vi "get_voltages.vi"(8 "error in (no error)":errorcluster, 11 "TrajectoryAK101022Resonance in":refnum<class "TrajectoryAK101022Resonance.lvclass">) -> (0 "error out":errorcluster, 1 "Vz min(V)":dbl, 2 "Vz max(V)":dbl, 3 "TrajectoryAK101022Resonance out":refnum<class "TrajectoryAK101022Resonance.lvclass">, 4 "Vy max(V)":dbl, 6 "Vy min(V)":dbl)   [LabVIEW 2010, in "TrajectoryAK101022Resonance.lvclass"]
uses:
  TrajectoryAK101022Resonance.lvclass
  TrajectoryAK101022Resonance.lvclass/TrajectoryAK101022Resonance.ctl
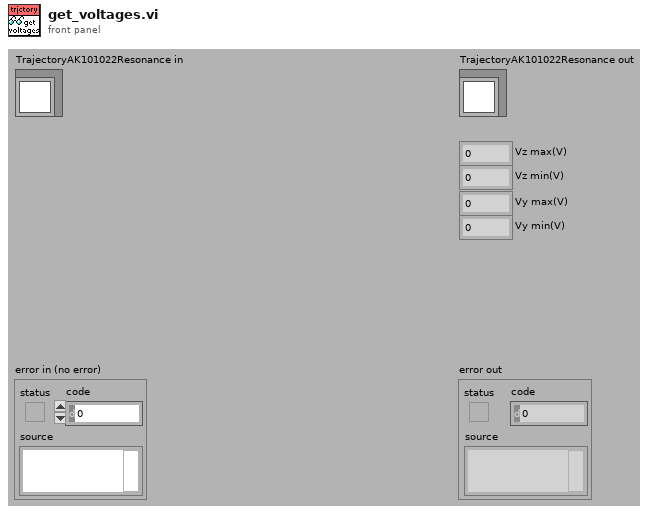
[diagram p1: front panel]
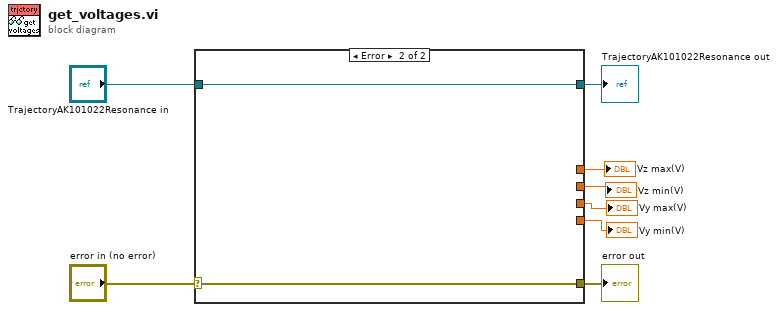
[diagram p0: block diagram]
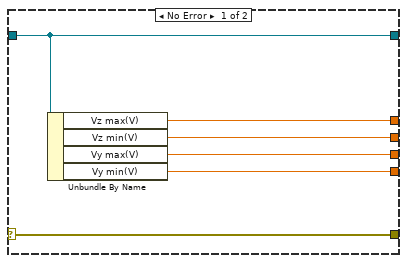
[diagram p2: hidden frame]
diagram:
  n1 = case shown="Error" "error in (no error)" {
    selector: "error in (no error)" -> [w14 w15]
    tunnel: [w14 w15] -> w7
    tunnel: [w13 w16] -> w5
    tunnel: "TrajectoryAK101022Resonance in" -> [w13 w16]
    tunnel: [w12 _] -> w4
    tunnel: [w11 _] -> w3
    tunnel: [w10 _] -> w2
    tunnel: [w9 _] -> w1
    frame No Error {
      n2 = Unbundle By Name(w13) -> ("Vz max(V)"=w12:dbl, "Vz min(V)"=w10:dbl, "Vy max(V)"=w9:dbl, "Vy min(V)"=w11:dbl)
    }
    frame Error {
    }
  }
  "error out" <- w7
  "TrajectoryAK101022Resonance out" <- w5
  "Vz max(V)" <- w4
  "Vz min(V)" <- w2
  "Vy max(V)" <- w1
  "Vy min(V)" <- w3
